vi "Read and deallocate string.vi"(8 "error in (no error)":errorcluster, 10 "string_len":u32, 11 "string_ptr":u64) -> (0 "error out":errorcluster, 3 "string":string)   [LabVIEW 2021, in "TOML2JSON.lvlib"]
uses:
  TOML2JSON.lvlib
  <vilib>/Utility/error.llb/Clear Errors.vi
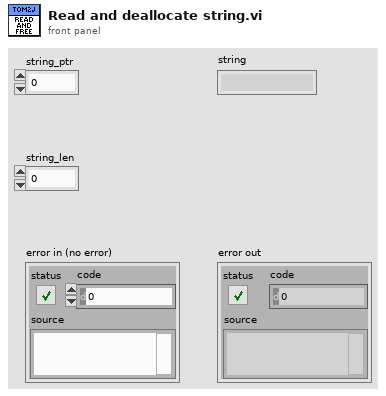
[diagram p1: front panel]
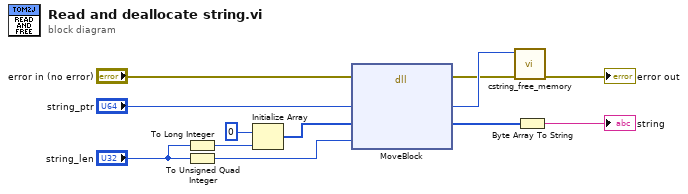
[diagram p0: block diagram]
diagram:
  n1 = To Long Integer(number="string_len") -> (32bit integer=w6:i32)
  n2 = To Unsigned Quad Integer(1:"string_len") -> (0:w4:u64)
  n3 = Initialize Array(u8 0, w6) -> (w5:u8[])
  n4 = dll-call lib="LabVIEW" fn="MoveBlock"(error in="error in (no error)", "src"="string_ptr", "dst"=w5, "size"=w4) -> (error out=w1:errorcluster, "src"=w2:u64, "dst"=w3:u8[])  [unwired: 4 in, 1 out]
  n5 = call "cstring_free_memory.vi"("error in (no error)"=w1, "ptr"=w2) -> ("error out"=→"error out":errorcluster)  [unwired: 9 in]
  n6 = Byte Array To String(unsigned byte array=w3) -> (string=→"string":string)
